vi "CreateLogFile.vi"(11 "Error In":errorcluster) -> (4 "EventDataOut":T1, 15 "Error Out":errorcluster)   [LabVIEW 2021, in "Event Logger.lvlib"]
uses:
  Event Logger.lvlib
  TypeDef/EventDataCluster.ctl
  TypeDef/EventValues.ctl
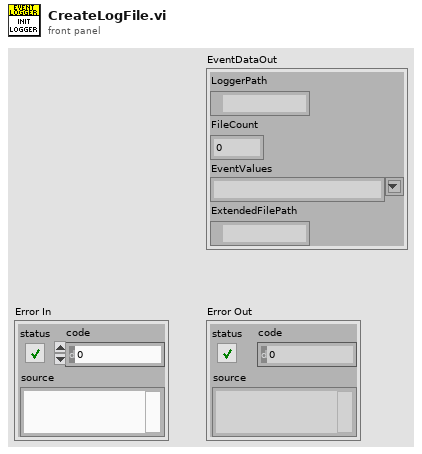
[diagram p1: front panel]
types:
  T1 = typedef "Event Logger.lvlib/EventDataCluster.ctl" = cluster{"LoggerPath":path, "FileCount":i32, "EventValues":T2, "ExtendedFilePath":path}
  T2 = typedef "Event Logger.lvlib/EventValues.ctl" = string
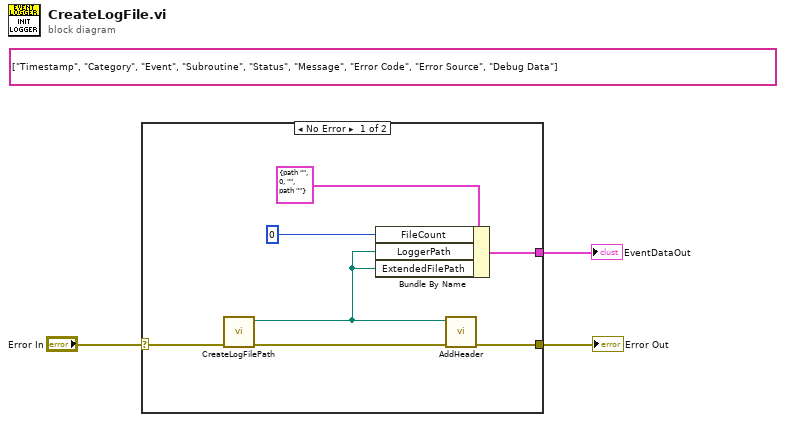
[diagram p0: block diagram]
diagram:
  (unwired) string[][] [["Timestamp", "Category", "Event", "Subroutine", "Status", "Message", "Error Code", "Error Source", "Debug Data"]] ("string")
  n1 = case shown="No Error" "Error In" {
    selector: "Error In" -> [w10 w11]
    tunnel: [w9 w11] -> w2
    tunnel: [w5 _] -> w1
    frame No Error {
      n2 = call "CreateLogFilePath.vi"("error in (no error)"=w10) -> ("error out"=w7:errorcluster, "LoggerPath"=w4:path)  [unwired: 9 in]
      n3 = Bundle By Name(cluster=T1 {"LoggerPath"=path "", "FileCount"=0, "EventValues"="", "ExtendedFilePath"=path ""} ("EventData"), "FileCount"=0, "LoggerPath"=w4, "ExtendedFilePath"=w4) -> (w5:T1)
      n4 = call "AddHeader.vi"("error in (no error)"=w7, "LoggerPath"=w4) -> ("error out"=w9:errorcluster)  [unwired: 9 in]
    }
    frame Error {
    }
  }
  "Error Out" <- w2
  "EventDataOut" <- w1
